vi "Begin.vi"(11 "Image Size":T5=enum."160x120") -> (0 "error out":errorcluster)   [LabVIEW 2012]
doc: "Called before other user functions, this VI is expected to open initial I/O refnums, load in file data, and do all program initialization. Notice that the <B>error out</B> terminal is simply used for data flow. Wiring it to other structures or subVIs ensures that this VI runs first."
uses:
  <vilib>/Rock Robotics/WPI/Camera/WPI_CameraImageSize.ctl
  <vilib>/Rock Robotics/SystemInterfaces/DIO/FPGA_DIOChannel.ctl
  <vilib>/Rock Robotics/WPI/Encoder/WPI_EncoderType.ctl
  <vilib>/Rock Robotics/SystemInterfaces/Typedef/FPGA_TypedefDigitalModule.ctl
  <vilib>/Rock Robotics/SystemInterfaces/DIO/FPGA_DIOPWMChannel.ctl
  <vilib>/Rock Robotics/WPI/Camera/WPI_CameraWhite Balance Values.ctl
  <vilib>/Rock Robotics/WPI/Camera/WPI_CameraExposure Values.ctl
  <vilib>/Rock Robotics/WPI/Camera/WPI_CameraFrameRate.ctl
  <vilib>/Rock Robotics/WPI/SafetyOutput/WPI_SafetyOutputConfigMenu.ctl
  <vilib>/Rock Robotics/WPI/DriverStation/WPI_DriverStationRobotMode2.ctl
  <vilib>/Rock Robotics/WPI/Joystick/WPI_JoystickDeviceEnum.ctl
  <vilib>/Rock Robotics/SystemInterfaces/DIO/FPGA_DIORelayChannel.ctl
  <vilib>/Rock Robotics/WPI/Solenoid/WPI_SolenoidChannel.ctl
  <vilib>/Rock Robotics/WPI/RobotDrive/WPI_RobotDriveOpen2MotorWithTalon.vi
  Robot Global Data.vi
  <vilib>/Rock Robotics/WPI/Solenoid/WPI_SolenoidOpenDouble.vi
  <vilib>/Rock Robotics/WPI/Counter/WPI_CounterDigitalInputToDigitalSource.vi
  <vilib>/Rock Robotics/WPI/MotorControl/WPI_MotorControlOpen Victor.vi
  <vilib>/Rock Robotics/WPI/Compressor/WPI_CompressorGetSetRefNum.vi
panel:
  in  "Wheel diameter (in)":dbl=6.0
  in  "Motor PWM Channel":T1
  in  "DIO Module":T2
  in  "Number Samples to Average":u8=1 min=1 max=128
  in  "Invert Direction":bool
  in  "Decoding Type":T3=enum."4x"
  in  "DistancePerCount (deg)":dbl=0.288
  in  "Encoder B Channel":T4=enum."DIO 2"
  in  "Encoder A Channel":T4
  in  "Minimum Rate":dbl=20.0
  out "Encoder Direction":string
  out "Encoder Alarm Status":string
  in  "Reset Encoder?":bool
  in  "Stop":bool
  out "Encoder Rate (deg/sec)":dbl
  in  "Motor Speed (-1 to 1)":dbl(slide) scale=-1.0..1.0
  out "Revolutions":dbl
  out "Distance (in)":dbl
  out "Current angle (deg)":dbl(knob) scale=0.0..360.0
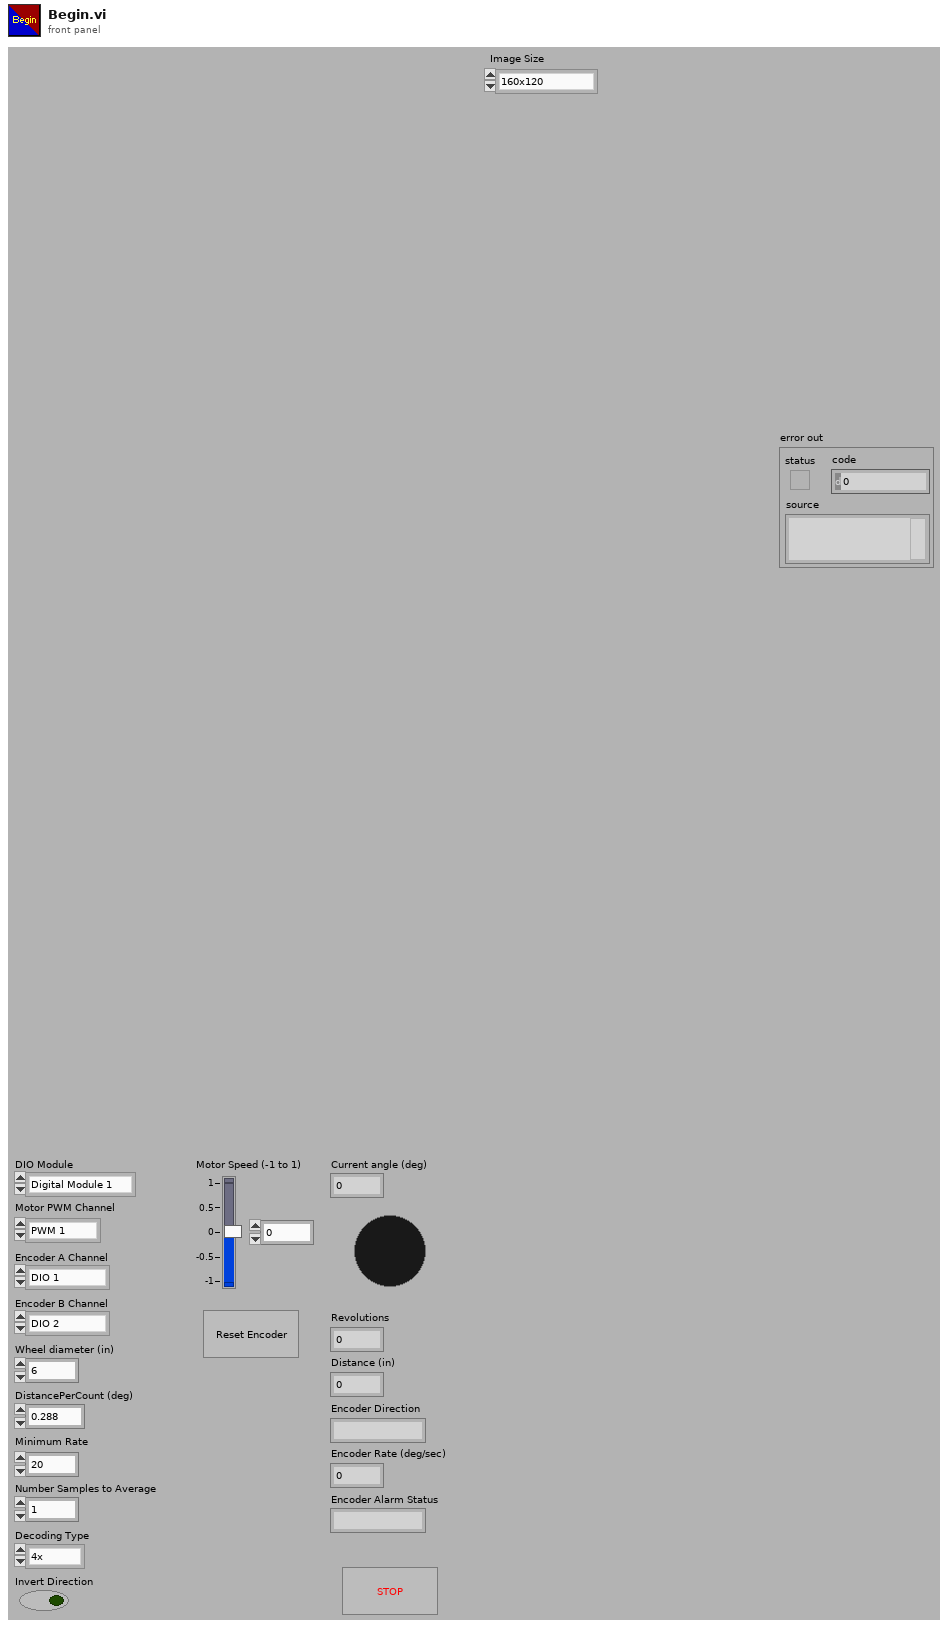
[diagram p1: front panel]
types:
  T1 = typedef "FPGA_DIOPWMChannel.ctl" = enum8{"PWM 1", "PWM 2", "PWM 3", "PWM 4", "PWM 5", "PWM 6", "PWM 7", "PWM 8", "PWM 9", "PWM 10", "Invalid"}
  T2 = typedef "FPGA_TypedefDigitalModule.ctl" = enum16{"Digital Module 1", "Digital Module 2"}
  T3 = typedef "WPI_EncoderType.ctl" = enum16{"1x", "2x", "4x"}
  T4 = typedef "FPGA_DIOChannel.ctl" = enum8{"DIO 1", "DIO 2", "DIO 3", "DIO 4", "DIO 5", "DIO 6", "DIO 7", "DIO 8", "DIO 9", "DIO 10", "DIO 11", "DIO 12", "DIO 13", "DIO 14", "Invalid"}
  T5 = typedef "WPI_CameraImageSize.ctl" = enum16{"640x480", "320x240", "160x120"}
  T6 = typedef "WPI_SolenoidChannel.ctl" = enum8{"Solenoid 1", "Solenoid 2", "Solenoid 3", "Solenoid 4", "Solenoid 5", "Solenoid 6", "Solenoid 7", "Solenoid 8", "Invalid"}
  T7 = typedef "FPGA_DIORelayChannel.ctl" = enum8{"Relay 1", "Relay 2", "Relay 3", "Relay 4", "Relay 5", "Relay 6", "Relay 7", "Relay 8", "Invalid"}
  T8 = typedef "WPI_JoystickDeviceEnum.ctl" = enum16{"USB 1", "USB 2", "USB 3", "USB 4", "Kinect 1", "Kinect 2"}
  T9 = typedef "WPI_DriverStationRobotMode2.ctl" = enum16{"Autonomous Disabled", "Autonomous Enabled", "Teleop Disabled", "Teleop Enabled", "Timeout", "Finish", "Test Disabled", "Test Enabled"}
  T10 = typedef "WPI_SafetyOutputConfigMenu.ctl" = enum16{"Enable", "Disable"}
  T11 = typedef "WPI_CameraFrameRate.ctl" = u32
  T12 = typedef "WPI_CameraExposure Values.ctl" = enum16{"Auto", "Flicker-free 50 Hz", "Flicker-free 60 Hz", "Hold current"}
  T13 = typedef "WPI_CameraWhite Balance Values.ctl" = enum16{"Auto", "Fixed indoor", "Fixed outdoor 1", "Fixed outdoor 2", "Fixed fluorescent 1", "Fixed fluorescent 2", "Hold current"}
  T14 = typedef "WPI_JoystickDevRef.ctl" = cluster{"Device":T8}
  T15 = typedef "WPI_RobotDriveDevRef.ctl" = cluster{"DevStatus":errorcluster, "Motors[]":T16[], "Square Inputs":bool, "Max Output":dbl, "Isochronous":bool}
  T16 = typedef "WPI_MotorControlDeviceRef.ctl" = cluster{"DeviceStatus":errorcluster, "Type":enum16{"PWM", "CAN"}, "PWM":cluster{"Digital Module":T2, "PWM Channel":T1, "DeadBand":T17}, "CAN":cluster{"Device Number":u8, "Control Mode":T18, "Semaphore":T19, "Max Vout":dbl}, "Invert":bool, "TransformRef":T20, "InvTransformRef":T20}
  T17 = typedef "WPI_PWMDeadband.ctl" = cluster{"Name":string, "maxPositivePwm":i32, "minPositivePwm":i32, "centerPwm":i32, "maxNegativePwm":i32, "minNegativePwm":i32, "angularRange":u16}
  T18 = typedef "WPI_CANJaguar_ControlMode.ctl" = enum8{"Percent VBus", "Current", "Speed", "Position", "Voltage"}
  T19 = typedef "Semaphore RefNum" = refnum<k1>
  T20 = typedef "WPI_PWMTransform_ConPane.ctl" = refnum<vi>
  T21 = typedef "WPI_CompressorDevRef.ctl" = cluster{"DevStatus":errorcluster, "DigitalInputDevRef":T22, "RelayDevRef":T23}
  T22 = typedef "WPI_DigitalInputDevRef.ctl" = cluster{"DevStatus":errorcluster, "DIO Channel":T4, "Digital Module":T2}
  T23 = typedef "WPI_RelayDevRef.ctl" = cluster{"DevStatus":errorcluster, "Relay Channel":T7, "Digital Module":T2, "Relay Direction":T24}
  T24 = typedef "WPI_RelayDirection.ctl" = enum16{"Both directions", "Forward only", "Reverse only"}
  T25 = typedef "WPI_CameraDevRef.ctl" = cluster{"Camera Address":string, "CameraStatus":errorcluster, "Acquire Image Notifier":refnum<notifier>}
  T26 = typedef "FPGA_CounterEncoderSourceConvertionLVSourceType.ctl" = cluster{"DevStatus":errorcluster, "AnalogTriggerMode?":bool, "DigitalMode":cluster{"Digital Module":T2, "DIO Channel":T27}, "AnalogTriggerMode":cluster{"AnalogTriggerIndex":T28, "OutputType":T29}}
  T27 = typedef "FPGA_DIODigitalSourceChannel.ctl" = enum8{"DIO 1", "DIO 2", "DIO 3", "DIO 4", "DIO 5", "DIO 6", "DIO 7", "DIO 8", "DIO 9", "DIO 10", "DIO 11", "DIO 12", "DIO 13", "DIO 14", "Disabled"}
  T28 = typedef "FPGA_AnalogTriggerIndex.ctl" = enum8{"Trig 0", "Trig 1", "Trig 2", "Trig 3", "Trig 4", "Trig 5", "Trig 6", "Trig 7", "Invalid"}
  T29 = typedef "FPGA_AnalogTriggerOutType.ctl" = enum16{"InWindow", "TriggerState", "Rising", "Falling"}
  T30 = typedef "WPI_EncoderDevRef.ctl" = cluster{"DevStatus":errorcluster, "EncoderIndex":T31, "CounterIndex":T32, "DistancePerCount":dbl, "Decoding Type":T3}
  T31 = typedef "FPGA_EncoderIdx.ctl" = enum8{"Enc 0", "Enc 1", "Enc 2", "Enc 3", "Invalid"}
  T32 = typedef "FPGA_CounterCtrSystemIndex.ctl" = enum8{"Ctr 0", "Ctr 1", "Ctr 2", "Ctr 3", "Ctr 4", "Ctr 5", "Ctr 6", "Ctr 7", "Invalid"}
  T33 = typedef "WPI_SolenoidDevRef.ctl" = cluster{"DevStatus":errorcluster, "Solenoid Module":T34, "Forward Solenoid Channel":T6, "Reverse Solenoid Channel":T6}
  T34 = typedef "FPGA_TypedefSolenoidModule.ctl" = enum16{"Solenoid Module 1", "Solenoid Module 2"}
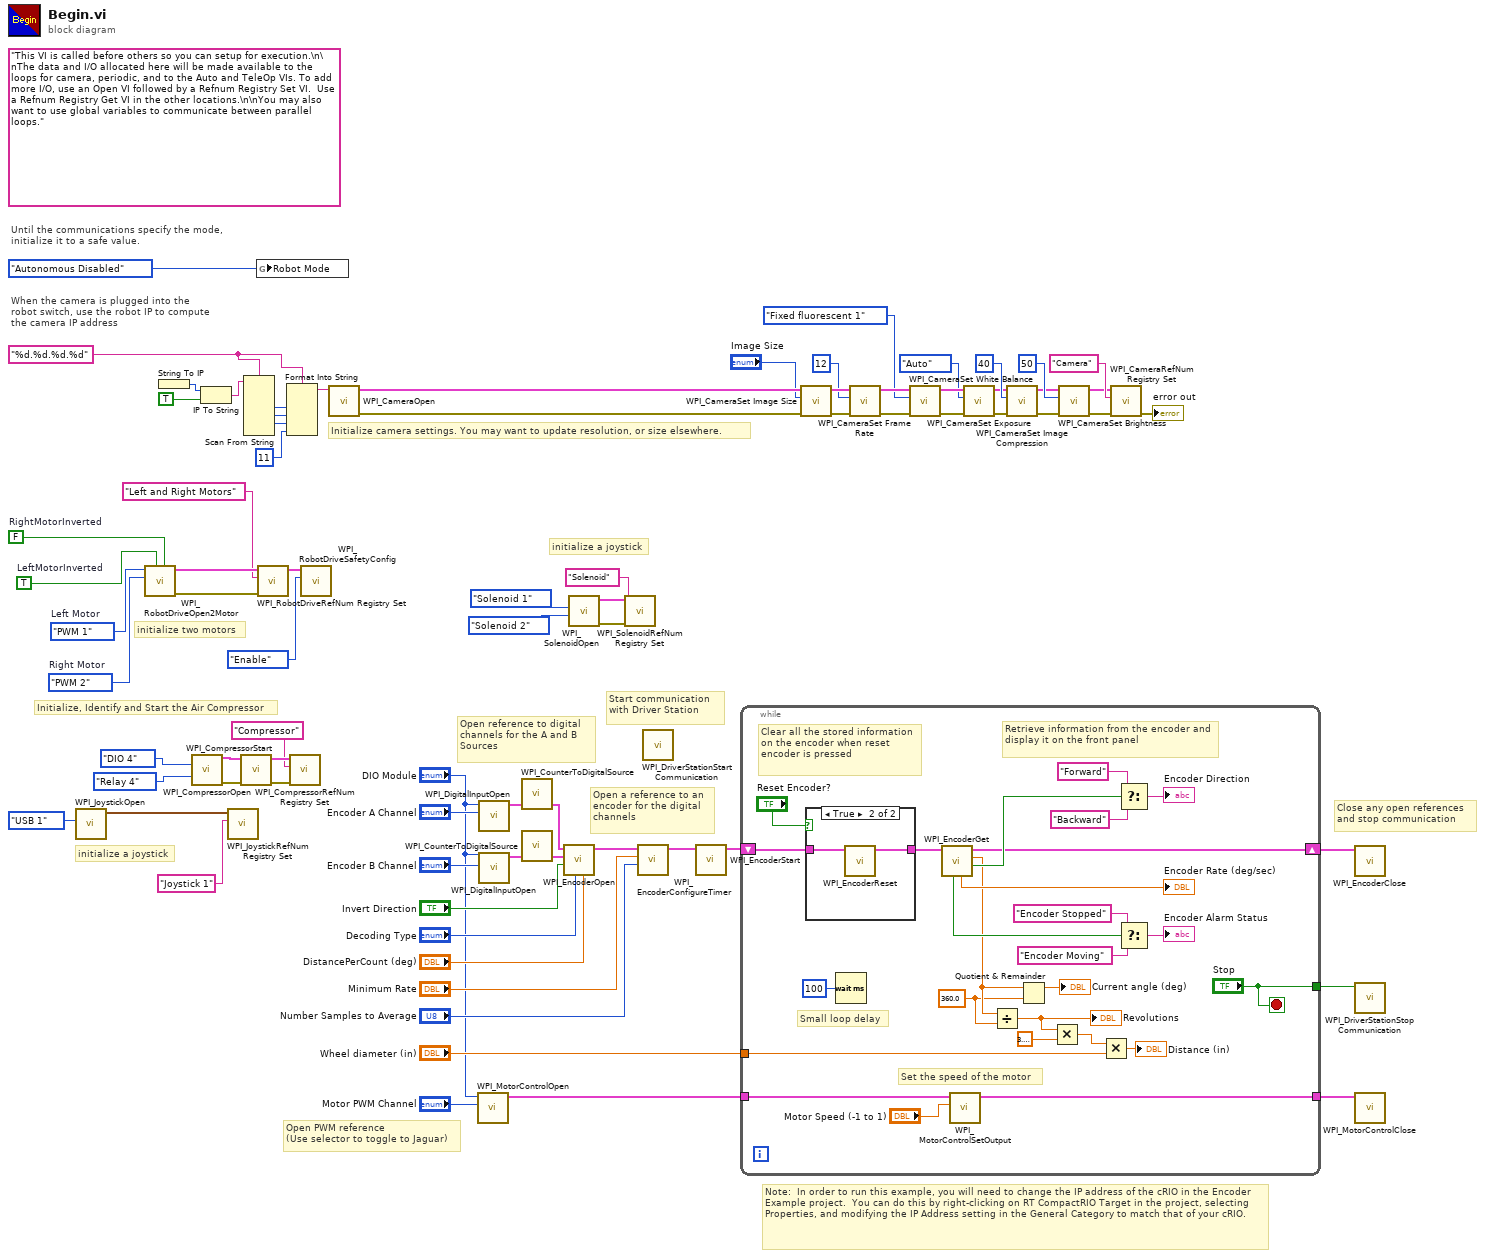
[diagram p0: block diagram]
diagram:
  w42 = "%d.%d.%d.%d" ("format string")
  (unwired) "This VI is called before others so you can setup for execution.\n\nThe data and I/O allocated here will be made available to the loops for camera, periodic, and to the Auto and TeleOp VIs. To add more I/O, use an Open VI followed by a Refnum Registry Set VI.  Use a Refnum Registry Get VI in the other locations.\n\nYou may also want to use global variables to communicate between parallel loops."
  w53 = FPGA_DIOPWMChannel."PWM 2"  # Right Motor
  w54 = FPGA_DIOPWMChannel."PWM 1"  # Left Motor
  w76 = TRUE  # LeftMotorInverted
  w77 = FALSE  # RightMotorInverted
  # "Open PWM reference\n(Use selector to toggle to Jaguar)"
  # "Start communication with Driver Station"
  # "Note:  In order to run this example, you will need to change the IP address of the cRIO in the Encoder Example project.  You can do this by right-clicking on RT CompactRIO Target in the project, selecting Properties, and modifying the IP Address setting in the General Category to match that of your cRIO."
  # "Close any open references\nand stop communication"
  # "Open a reference to an\nencoder for the digital \nchannels"
  # "Open reference to digital \nchannels for the A and B\nSources"
  # "initialize a joystick"
  # "Initialize, Identify and Start the Air Compressor"
  # "initialize a joystick"
  # "Until the communications specify the mode,\ninitialize it to a safe value."
  # "When the camera is plugged into the\nrobot switch, use the robot IP to compute\nthe camera IP address"
  # "initialize two motors"
  # "Initialize camera settings. You may want to update resolution, or size elsewhere."
  n1 = call <vilib>:"WPI_JoystickOpen.vi"("JoystickDevice"=WPI_JoystickDeviceEnum."USB 1") -> ("JoystickDevRef"=w36:T14)  [unwired: 10 in]
  n2 = call-poly <vilib>:"WPI_RobotDriveOpen2Motor.vi"("Right Motor Inverted"=w77, "Left Motor Inverted"=w76, "Right Motor"=w53, "Left Motor"=w54) -> ("error out"=w72:errorcluster, "RobotDriveDevRef"=w74:T15)  [unwired: 1 in, 5 out]
  n3 = String To IP() -> (0:w49:u32)  [unwired: 1 in]
  n4 = call <vilib>:"WPI_CompressorOpen.vi"("Pressure Switch DIO Channel"=FPGA_DIOChannel."DIO 4", "Relay Channel"=FPGA_DIORelayChannel."Relay 4") -> ("CompressorDevRef"=w31:T21, "error out"=w30:errorcluster)  [unwired: 12 in]
  n5 = IP To String(1:TRUE ("dot notation? (F)"), 2:w49) -> (0:w47:string)
  n6 = call <vilib>:"WPI_JoystickRefNum Registry Set.vi"("refnum name"="Joystick 1", "JoystickDevRef"=w36) -> ()  [unwired: 8 in, 2 out]
  n7 = call <vilib>:"WPI_CompressorStart.vi"("error in (no error)"=w30, "CompressorDevRef"=w31) -> ("error out"=w33:errorcluster, "CompressorDevRef"=w32:T21)  [unwired: 8 in]
  n8 = Scan From String(format string=w42, input string=w47) -> (output 1=w46:i32, output 2=w45:i32, output 3=w44:i32)  [unwired: 7 in, 3 out]
  n9 = global write "Robot Global Data.vi" "Robot Mode"(WPI_DriverStationRobotMode2."Autonomous Disabled" ("Robot Mode")) -> ()
  n10 = call <vilib>:"WPI_RobotDriveRefNum Registry Set.vi"("error in (no error)"=w72, "refnum name"="Left and Right Motors", "RobotDriveDevRef"=w74) -> ("RobotDriveDevRef"=w41:T15)  [unwired: 8 out]
  n11 = Format Into String(format string=w42, w46, w45, w44, 11 ("Compression")) -> (resulting string=w38:string)  [unwired: 2 in, 1 out]
  n12 = call <vilib>:"WPI_CompressorRefNum Registry Set.vi"("error in (no error)"=w33, "refnum name"="Compressor", "CompressorDevRef"=w32) -> ()  [unwired: 8 in, 1 out]
  n13 = call <vilib>:"WPI_RobotDriveSafetyConfig.vi"("mode"=WPI_SafetyOutputConfigMenu."Enable", "RobotDriveDevRef"=w41) -> ()  [unwired: 8 in, 2 out]
  n14 = call <vilib>:"WPI_CameraOpen.vi"("Camera Address"=w38) -> ("error out"=w63:errorcluster, "CameraDevRef"=w64:T25)  [unwired: 1 in, 8 out]
  n15 = call-poly <vilib>:"WPI_MotorControlOpen.vi"("PWM Channel"="Motor PWM Channel", "Digital Module (Module 1)"="DIO Module") -> ("MotorControlDeviceRef"=w3:T16)  [unwired: 5 in, 4 out]
  n16 = call <vilib>:"WPI_DigitalInputOpen.vi"("DIO Channel"="Encoder A Channel", "Digital Module (Module 1)"="DIO Module") -> ("DigitalInputDevRef"=w16:T22)  [unwired: 1 in, 8 out]
  n17 = call <vilib>:"WPI_DigitalInputOpen.vi"("DIO Channel"="Encoder B Channel", "Digital Module (Module 1)"="DIO Module") -> ("DigitalInputDevRef"=w17:T22)  [unwired: 1 in, 8 out]
  n18 = call-poly <vilib>:"WPI_CounterToDigitalSource.vi"("DigitalInputDevRef"=w16) -> ("Digital Source"=w15:T26)  [unwired: 6 out]
  n19 = call-poly <vilib>:"WPI_CounterToDigitalSource.vi"("DigitalInputDevRef"=w17) -> ("Digital Source"=w18:T26)  [unwired: 6 out]
  n20 = call <vilib>:"WPI_EncoderOpen.vi"("DistancePerCount"="DistancePerCount (deg)", "Decoding Type"="Decoding Type", "Invert Direction (False)"="Invert Direction", "BSource"=w18, "ASource"=w15) -> ("EncoderDevRef"=w8:T30)  [unwired: 3 in, 3 out]
  n21 = call-poly <vilib>:"WPI_SolenoidOpen.vi"("Reverse Solenoid Channel"=WPI_SolenoidChannel."Solenoid 2", "Forward Solenoid Channel"=WPI_SolenoidChannel."Solenoid 1") -> ("error out"=w24:errorcluster, "SolenoidDevRef"=w23:T33)  [unwired: 8 in]
  n22 = call <vilib>:"WPI_SolenoidRefNum Registry Set.vi"("error in (no error)"=w24, "refnum name"="Solenoid", "SolenoidDevRef"=w23) -> ()  [unwired: 7 in, 2 out]
  n23 = call <vilib>:"WPI_EncoderConfigureTimer.vi"("Number Samples to Average"="Number Samples to Average", "Minimum Rate"="Minimum Rate", "EncoderDevRef"=w8) -> ("EncoderDevRef"=w9:T30)  [unwired: 1 in, 7 out]
  n24 = call <vilib>:"WPI_DriverStationStart Communication.vi"() -> ()  [unwired: 1 in, 11 out]
  n25 = call <vilib>:"WPI_EncoderStart.vi"("EncoderDevRef"=w9) -> ("EncoderDevRef"=w21:T30)  [unwired: 1 in, 9 out]
  n26 = while {
    shift-right: [w96] -> w20
    shift-left: w21 -> [w101]
    tunnel: ["Stop"] -> w19
    tunnel: w3 -> [w89]
    tunnel: [w88] -> w5
    tunnel: "Wheel diameter (in)" -> [w83]
    stop <- "Stop" stop-if-true
    w86 = 360.0 ("y")
    # "Retrieve information from the encoder and display it on the front panel"
    # "Set the speed of the motor"
    # "Small loop delay"
    # "Clear all the stored information on the encoder when reset encoder is pressed"
    n27 = case shown="True" "Reset Encoder?" {
      tunnel: w101 -> [w104 w106]
      tunnel: [w104 w105] -> w99
      frame False {
      }
      frame True {
        n28 = call <vilib>:"WPI_EncoderReset.vi"("EncoderDevRef"=w106) -> ("EncoderDevRef"=w105:T30)  [unwired: 1 in, 9 out]
      }
    }
    n29 = Wait (ms)(milliseconds to wait=u32 100) -> ()  [unwired: 1 out]
    n30 = call <vilib>:"WPI_EncoderGet.vi"("EncoderDevRef"=w99) -> ("Direction"=w98:bool, "Distance"=w87:dbl, "EncoderDevRef"=w96:T30, "Rate"=→"Encoder Rate (deg/sec)":dbl, "Stopped"=w97:bool)  [unwired: 1 in, 5 out]
    n31 = call <vilib>:"WPI_MotorControlSetOutput.vi"("Output"="Motor Speed (-1 to 1)", "MotorControlDevRef"=w89) -> ("MotorControlDevRef"=w88:T16)  [unwired: 3 in, 6 out]
    n32 = Divide(x=w87, y=w86) -> (x/y=w85:dbl)
    "Revolutions" <- w85
    n33 = Quotient & Remainder(x=w87, y=w86) -> (x-y*floor(x/y)=→"Current angle (deg)":dbl)  [unwired: 1 out]
    n34 = Multiply(x=w85, y=3.141592653589793) -> (x*y=w81:dbl)
    n35 = Multiply(x=w81, y=w83) -> (x*y=→"Distance (in)":dbl)
    n36 = Select(t="Forward", s=w98, f="Backward") -> (s? t:f=→"Encoder Direction":string)
    n37 = Select(t="Encoder Stopped", s=w97, f="Encoder Moving") -> (s? t:f=→"Encoder Alarm Status":string)
  }
  n38 = call <vilib>:"WPI_CameraSet Image Size.vi"("error in (no error)"=w63, "Image Size"="Image Size", "CameraDevRef"=w64) -> ("error out"=w62:errorcluster, "CameraDevRef Out"=w65:T25)  [unwired: 7 out]
  n39 = call <vilib>:"WPI_CameraSet Frame Rate.vi"("error in (no error)"=w62, "Frame Rate (fps)"=T11 12, "CameraDevRef"=w65) -> ("error out"=w61:errorcluster, "CameraDevRef Out"=w67:T25)  [unwired: 7 out]
  n40 = call <vilib>:"WPI_CameraSet White Balance.vi"("error in (no error)"=w61, "White Balance"=WPI_CameraWhite_Balance_Values."Fixed fluorescent 1", "CameraDevRef"=w67) -> ("error out"=w60:errorcluster, "CameraDevRef Out"=w66:T25)  [unwired: 7 out]
  n41 = call <vilib>:"WPI_CameraSet Exposure.vi"("error in (no error)"=w60, "Exposure"=WPI_CameraExposure_Values."Auto", "CameraDevRef"=w66) -> ("error out"=w59:errorcluster, "CameraDevRef Out"=w69:T25)  [unwired: 7 out]
  n42 = call <vilib>:"WPI_CameraSet Image Compression.vi"("error in (no error)"=w59, "Compression"=40, "CameraDevRef"=w69) -> ("error out"=w58:errorcluster, "CameraDevRef Out"=w68:T25)  [unwired: 7 out]
  n43 = call <vilib>:"WPI_CameraSet Brightness.vi"("error in (no error)"=w58, "Brightness"=50, "CameraDevRef"=w68) -> ("error out"=w56:errorcluster, "CameraDevRef Out"=w57:T25)  [unwired: 7 out]
  n44 = call <vilib>:"WPI_CameraRefNum Registry Set.vi"("error in (no error)"=w56, "refnum name"="Camera", "CameraDevRef"=w57) -> ("error out"=→"error out":errorcluster)  [unwired: 8 out]
  n45 = call <vilib>:"WPI_EncoderClose.vi"("EncoderDevRef"=w20) -> ()  [unwired: 2 in, 9 out]
  n46 = call <vilib>:"WPI_DriverStationStop Communication.vi"("StopCommunication"=w19) -> ()  [unwired: 1 in, 10 out]
  n47 = call <vilib>:"WPI_MotorControlClose.vi"("MotorControlDevRef"=w5) -> ()  [unwired: 1 in, 10 out]
